vi "Enviar producto.vi"(8 "error in (no error)":errorcluster, 9 "index":u16, 10 "Item names":string[][](array[string]), 11 "LHL Actor in":refnum<class "LHL Actor.lvclass">) -> (0 "error out":errorcluster, 3 "LHL Actor out":refnum<class "LHL Actor.lvclass">)   [LabVIEW 2020, in "LHL Actor.lvlib" / "LHL Actor.lvclass"]
uses:
  LHL Actor.lvclass
  C:/Program Files/National Instruments/LabVIEW 2020/vi.lib/ActorFramework/Actor/Actor.lvclass
  LHL Actor.lvclass/LHL Actor.ctl
  <vilib>/ActorFramework/Actor/Actor.lvclass/Actor.ctl
  UI Actor Messages/Compra Msg/Compra Msg.lvclass/Compra Msg.ctl
  <vilib>/ActorFramework/Message Enqueuer/Message Enqueuer.lvclass/Message Enqueuer.ctl
  <vilib>/ActorFramework/Message Enqueuer/Enqueue.vi
  UI Actor Messages/Compra Msg/Compra Msg.lvclass
  C:/Program Files/National Instruments/LabVIEW 2020/vi.lib/ActorFramework/Message/Message.lvclass
  <vilib>/ActorFramework/Message Priority Queue/Priority Enqueue.vi
  <vilib>/ActorFramework/Actor/Actor.lvclass
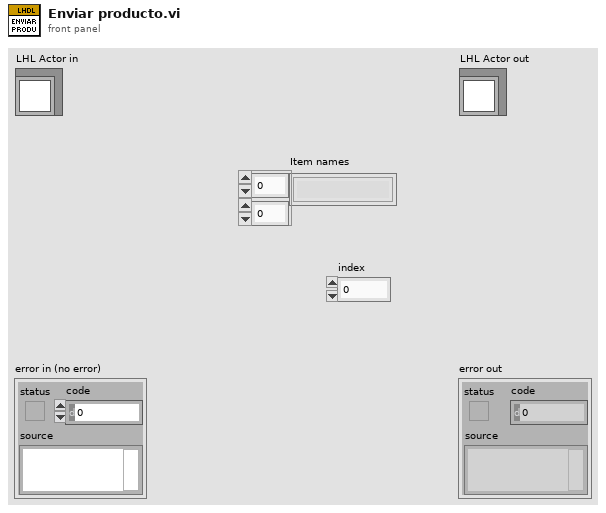
[diagram p1: front panel]
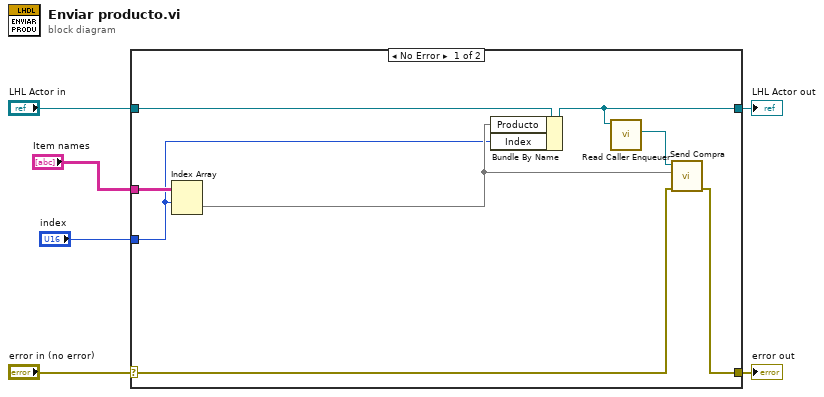
[diagram p0: block diagram]
diagram:
  n1 = case shown="No Error" "error in (no error)" {
    selector: "error in (no error)" -> [w9 w16]
    tunnel: [w8 w16] -> w5
    tunnel: [w12 w15] -> w3
    tunnel: "LHL Actor in" -> [w14 w15]
    tunnel: "Item names" -> [w13 _]
    tunnel: "index" -> [w7 _]
    frame No Error {
      n2 = Index Array "Index Array"(array=w13, index (row)=w7) -> (element=w10:string[])  [unwired: 1 in]
      n3 = Bundle By Name(cluster=w14, "Producto"=w10, "Index"=w7) -> (w12:refnum<class "LHL Actor.lvclass">)
      n4 = call <vilib>:"Read Caller Enqueuer.vi"("Actor"=w12) -> ("Caller Enqueuer"=w11:refnum<class "Message Enqueuer.lvclass">)  [unwired: 10 in]
      n5 = call "Send Compra.vi"("error in (no error)"=w9, "Producto"=w10, "Message Enqueuer"=w11) -> ("error out"=w8:errorcluster)  [unwired: 7 in, 1 out]
    }
    frame Error {
    }
  }
  "error out" <- w5
  "LHL Actor out" <- w3
